vi "test.reqwest_get.vi"() -> ()   [LabVIEW 2020]
uses:
  reqwest/reQwestClient.lvclass
panel:
  out "response_body":string
  in  "url":string
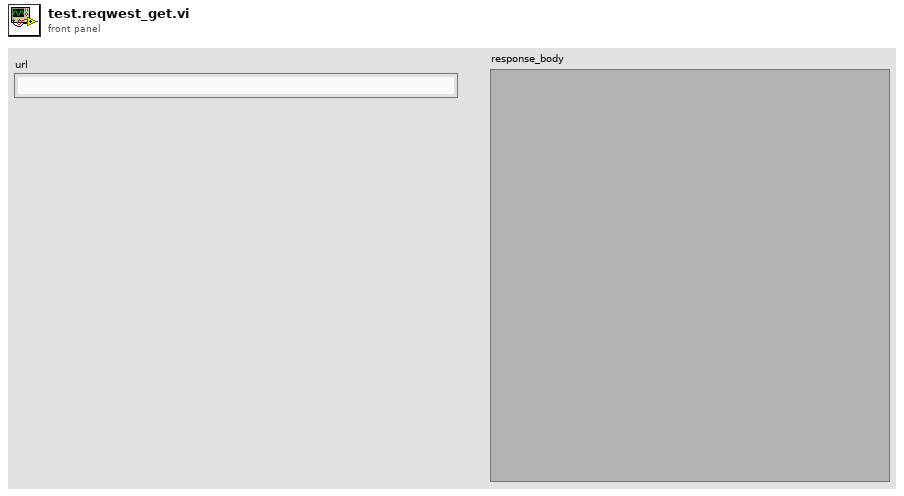
[diagram p1: front panel]
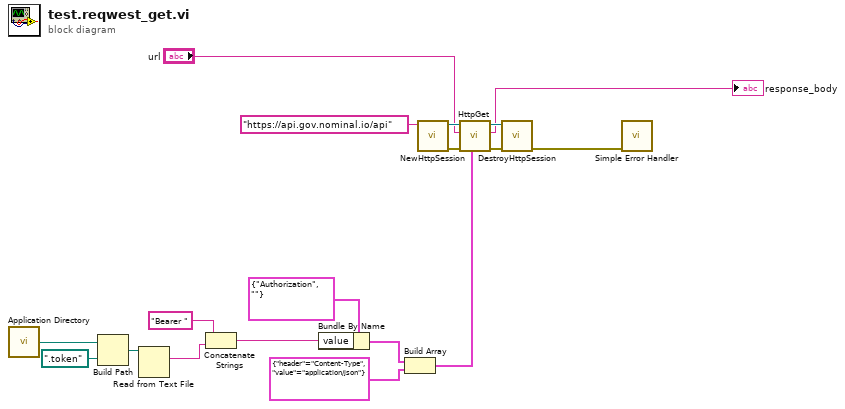
[diagram p0: block diagram]
diagram:
  n1 = call <vilib>:"Application Directory.vi"() -> ("Application Directory"=w8:path)
  n2 = Build Path(base path=w8, name or relative path=path ".token") -> (appended path=w6:path)
  n3 = Read from Text File(file (use dialog)=w6) -> (text=w5:string)  [unwired: 3 in, 3 out]
  n4 = Concatenate Strings("Bearer " ("value"), w5) -> (w12:string)
  n5 = Bundle By Name(cluster=cluster{"header":string, "value":string} {"header"="Authorization", "value"=""} ("Header"), "value"=w12) -> (w11:cluster{"header":string, "value":string})
  n6 = Build Array(w11, cluster{"header":string, "value":string} {"header"="Content-Type", "value"="application/json"} ("Header")) -> (w9:cluster{"header":string, "value":string}[])
  n7 = call "NewHttpSession.vi"("base url"="https://api.gov.nominal.io/api") -> ("error out"=w17:errorcluster, "reQwestClient"=w18:refnum<class "reQwestClient.lvclass">)  [unwired: 9 in]
  n8 = call "HttpGet.vi"("request specific headers"=w9, "error in"=w17, "url"="url", "reQwestClient in"=w18) -> ("error out"=w15:errorcluster, "response_body"=→"response_body":string, "reQwestClient out"=w16:refnum<class "reQwestClient.lvclass">)  [unwired: 5 in]
  n9 = call "DestroyHttpSession.vi"("error in"=w15, "reQwestClient in"=w16) -> ("error out"=w1:errorcluster)  [unwired: 9 in]
  n10 = call <vilib>:"Simple Error Handler.vi"("error in (no error)"=w1) -> ()  [unwired: 4 in, 5 out]
